vi "poly_control_value_from_name_self_single.vi"(8 "error in (no error)":errorcluster, 9 "control name":string) -> (0 "error out":errorcluster, 1 "Value":variant, 4 "found?":bool, 5 "ctrl ref":refnum<vi>)   [LabVIEW 2015]
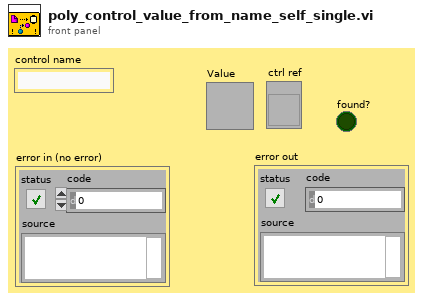
[diagram p1: front panel]
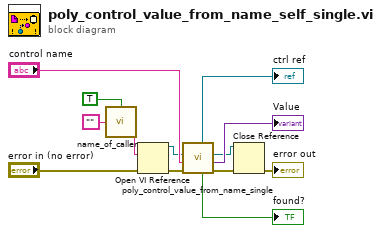
[diagram p0: block diagram]
diagram:
  n1 = call "name_of_caller.vi"("is in inlined vi? (F)"=TRUE, "name of caller in"="") -> ("name of caller out"=w8:string)  [unwired: 2 in]
  n2 = Open VI Reference(vi path=w8, error in (no error)="error in (no error)") -> (vi reference=w5:refnum<vi>, error out=w6:errorcluster)  [unwired: 4 in]
  n3 = call "poly_control_value_from_name_single.vi"("error in (no error)"=w6, "control name"="control name", "vi ref"=w5) -> ("error out"=w4:errorcluster, "Value"=→"Value":variant, "vi ref dup"=w2:refnum<vi>, "found?"=→"found?":bool, "ctrl ref"=→"ctrl ref":refnum<vi>)  [unwired: 4 in]
  n4 = Close Reference(reference=w2, error in (no error)=w4) -> (error out=→"error out":errorcluster)
